vi "Download File To Buffer.vi"(6 "timeout (ms)":i32=30000, 8 "error in":errorcluster, 10 "remote path":string, 11 "session in":refnum<class "Session.lvclass">) -> (0 "error out":errorcluster, 2 "buffer":u8[](array[numeric]), 3 "session out":refnum<class "Session.lvclass">)   [LabVIEW 2020, in "NI_SFTP.lvlib"]
doc: "Downloads a remote file, returning the contents as a byte array."
uses:
  <vilib>/net/SFTP/NI_SFTP.lvlib
  <vilib>/net/SFTP/Session/Session.lvclass
  <vilib>/net/SFTP/API/Support/Download/Buffer/Buffer Download Controller.lvclass
  <vilib>/Utility/Deadline/NI_Deadline.lvlib
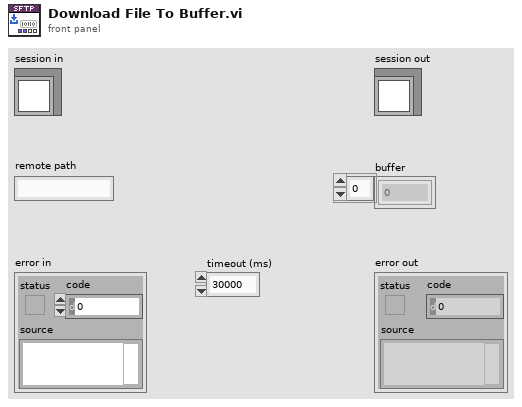
[diagram p1: front panel]
types:
  T1 = typedef "NI_Deadline.lvlib/Deadline.ctl" = cluster{"mode":T2, "deadline (ms)":u32}
  T2 = typedef "NI_Deadline.lvlib/Mode.ctl" = enum16{"Relative", "Use deadline", "Wait forever", "Nonblocking", "N/A"}
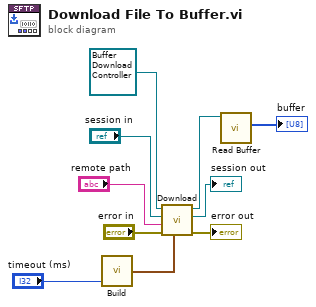
[diagram p0: block diagram]
diagram:
  n1 = call <vilib>:"Build.vi"("timeout (ms)"="timeout (ms)") -> ("Deadline out"=w1:T1)  [unwired: 2 in]
  n2 = call-dynamic "Download.vi"("deadline"=w1, "error in"="error in", "remote path"="remote path", "session in"="session in", "NI_SFTP.lvlib:Generic Download Controller.lvclass"=refnum<class "Buffer Download Controller.lvclass"> refnum ("NI_SFTP.lvlib:Buffer Download Controller.lvclass")) -> ("error out"=→"error out":errorcluster, "session out"=→"session out":refnum<class "Session.lvclass">, "NI_SFTP.lvlib:Generic Download Controller.lvclass 2"=w6:refnum<class "Buffer Download Controller.lvclass">)  [unwired: 4 in]
  n3 = call <vilib>:"Read Buffer.vi"("Buffer Download Controller in"=w6) -> ("buffer"=→"buffer":u8[])  [unwired: 9 in, 1 out]
